vi "System_ID.vi"() -> ()   [LabVIEW 2016]
uses:
  <vilib>/FPGAPlugInAG/myRIO-1900/niLvFpga_Open_myRIO-1900.vi
  <vilib>/rvi/interface/common/dynamic/niFpgaDynamicAddResources.vi
  <vilib>/Utility/error.llb/Error Cluster From Error Code.vi
  <vilib>/rvi/errors/niLvFpgaAdjustHostInterfaceError.vi
  <vilib>/FPGAPlugInAG/Dynamic/niLvFpga_Close_Dynamic.vi
  <vilib>/rvi/interface/nirviOpenFPGA/nirviOpenFPGA.xnode
  FPGA Bitfiles/SheepdogRobotPro_FPGATarget_RobotFPGAUtility_97tw+GI730k.lvbitx
  <vilib>/rvi/interface/nirviReadWriteControl/nirviReadWriteControl.xnode
  <vilib>/rvi/interface/nirviCloseFPGA/nirviCloseFPGA.xnode
  <vilib>/rvi/interface/Simulation/niFpgaSimulationCallBeginRW.vi
  NiFpgaLv.dll
panel:
  in  "PWM":dbl
  in  "stop":bool
  out "B":dbl(graph)
  out "A":dbl(graph)
  out "Wheel B Position":dbl
  out "Wheel B Speed":dbl
  out "Wheel A Position":dbl
  out "Wheel A Speed":dbl
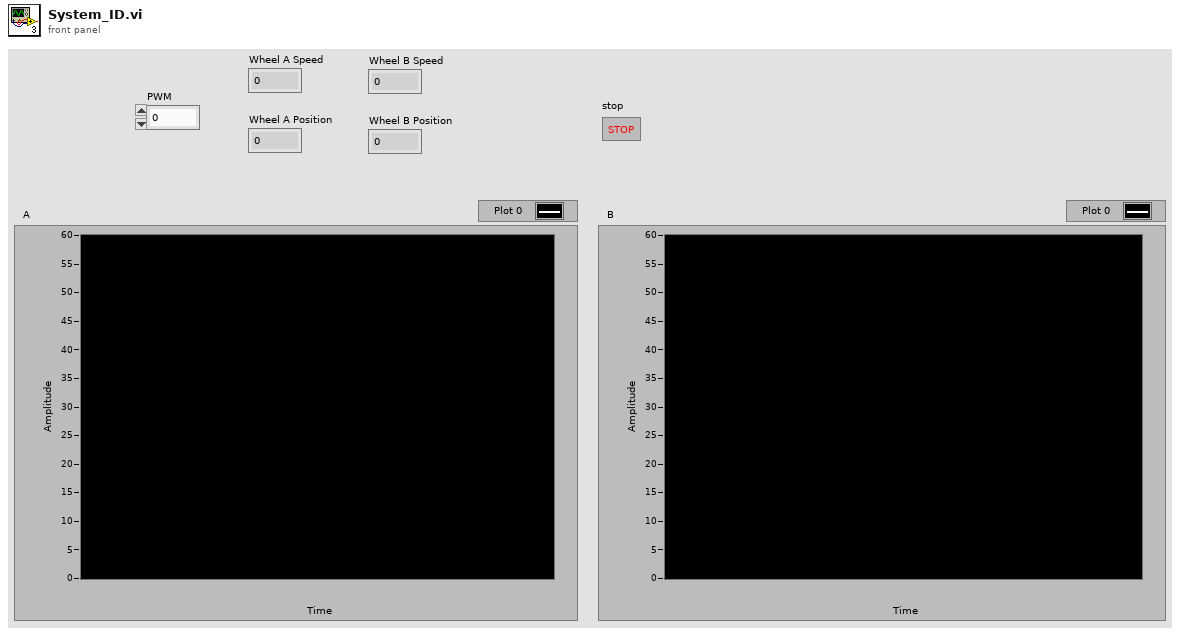
[diagram p1: front panel]
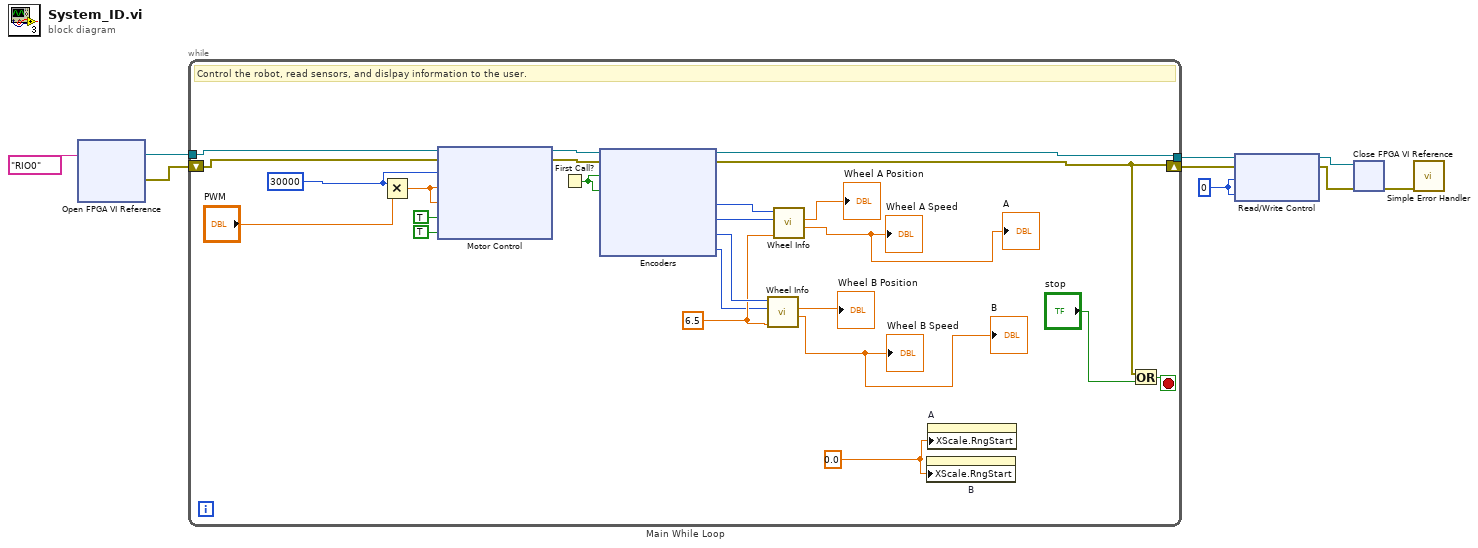
[diagram p0: block diagram]
diagram:
  w4 = 0
  n1 = xnode "Open FPGA VI Reference"("resource name"=tag "RIO0") -> ("FPGA VI Reference Out"=w7:refnum<k20>, "error out"=w8:errorcluster)  [unwired: 1 in]
  n2 = while "Main While Loop" {
    shift-right: [w31] -> w5
    shift-left: w8 -> [w27]
    tunnel: w7 -> [w24]
    tunnel: [w32] -> w6
    stop <- w33 stop-if-true
    w12 = 0.0
    w19 = 6.5
    w13 = 30000
    # "Control the robot, read sensors, and dislpay information to the user."
    n3 = Multiply(x=w13, y="PWM") -> (x*y=w28:dbl)
    n4 = xnode "Motor Control"("FPGA VI Reference In"=w24, "error in"=w27, "Duty Cycle Divisor"=w13, "Duty Cycle 1"=w28, "Duty Cycle 2"=w28, "Motor Dir 1"=TRUE, "Motor Dir 2"=TRUE) -> ("FPGA VI Reference Out"=w30:refnum<k20>, "error out"=w29:errorcluster)
    n5 = First Call?() -> (First Call?: T/F=w23:bool)
    n6 = xnode "Encoders"("FPGA VI Reference In"=w30, "error in"=w29, "Reset Encoder 1"=w23, "Reset Encoder 2"=w23) -> ("FPGA VI Reference Out"=w32:refnum<k20>, "error out"=w31:errorcluster, "Encoder 1 Position"=w22:i16, "Encoder 1 Period"=w21:u32, "Encoder 2 Position"=w20:i16, "Encoder 2 Period"=w10:u32)
    n7 = call "Wheel Info.vi"("Wheel Diameter"=w19, "Encoder Period"=w10, "Encoder Position"=w20) -> ("Wheel Speed"=→"Wheel B Speed" →"B":dbl, "Wheel Position"=→"Wheel B Position":dbl)  [unwired: 7 in]
    n8 = call "Wheel Info.vi"("Wheel Diameter"=w19, "Encoder Period"=w21, "Encoder Position"=w22) -> ("Wheel Speed"=→"Wheel A Speed" →"A":dbl, "Wheel Position"=→"Wheel A Position":dbl)  [unwired: 7 in]
    n9 = property on="B" class="WFChart (strict)"("XScale.RngStart"=w12) -> ()  [unwired: 2 in, 2 out]
    n10 = property on="A" class="WFChart (strict)"("XScale.RngStart"=w12) -> ()  [unwired: 2 in, 2 out]
    n11 = Or(x=w31, y="stop") -> (x .or. y?=w33:bool)
  }
  n12 = xnode "Read/Write Control"("FPGA VI Reference In"=w6, "error in"=w5, "Duty Cycle 1"=w4, "Duty Cycle 2"=w4) -> ("FPGA VI Reference Out"=w2:refnum<k20>, "error out"=w3:errorcluster)
  n13 = xnode "Close FPGA VI Reference"("FPGA VI Reference In"=w2, "error in"=w3) -> ("error out"=w1:errorcluster)
  n14 = call <vilib>:"Simple Error Handler.vi"("error in (no error)"=w1) -> ()  [unwired: 4 in, 5 out]
